vi "L298N stepper.vi"(2 "Baud Rate":u32=9600, 3 "Serial Port":refnum<visa-resource-name>) -> ()   [LabVIEW 2010]
uses:
  <vilib>/Instr/_visa.llb/VISA Set IO Buffer Mask.ctl
  <vilib>/Instr/_visa.llb/VISA Configure Serial Port (Instr).vi
panel:
  in  "stop":bool
  in  "Send":bool=TRUE
  out "Butes Written":u32
  out "X Step Position":i16
  out "String sent to Arduino":string
  in  "X Steps Setpoint":i16
  out "Status":errorcluster
  out "VISA resource\n name out":refnum<visa-resource-name>
  # "Serial Settings"
  # "Debug"
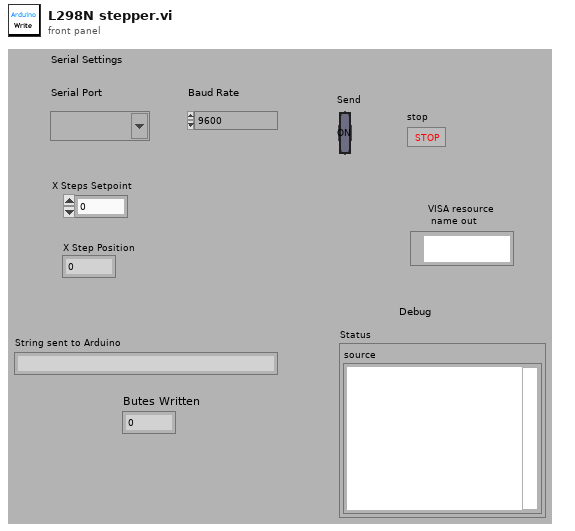
[diagram p1: front panel]
types:
  T1 = typedef "VISA Set IO Buffer Mask.ctl" = u16
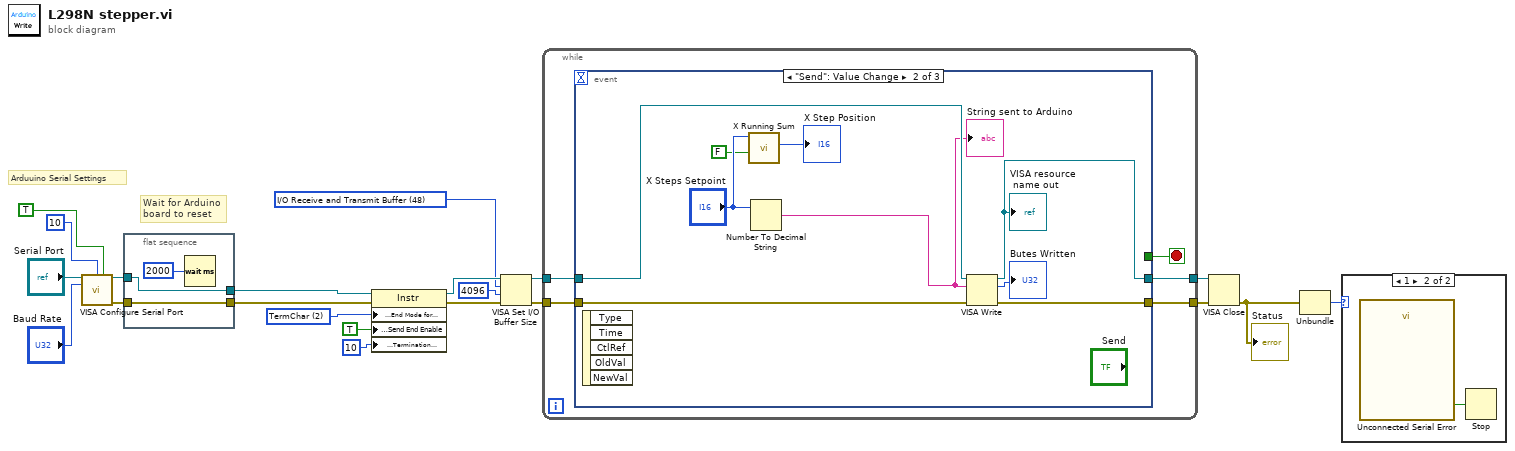
[diagram p0: block diagram]
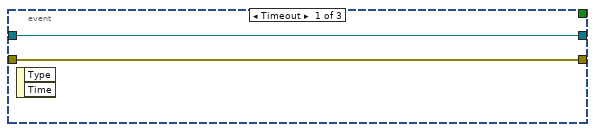
[diagram p2: hidden frame]
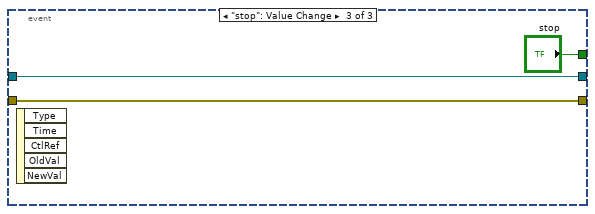
[diagram p3: hidden frame]
diagram:
  w7 = u16 2 items=["None", "Last Bit", "TermChar", "Break"] ("Serial Settings:End Mode for Writes")
  w5 = T1 48 items=["I/O Receive Buffer"=16, "I/O Transmit Buffer"=32, "I/O Receive and Transmit Buffer"=48] ("Mask")
  # "Wait for Arduino \nboard to reset"
  # "Arduuino Serial Settings"
  n1 = call-poly "VISA Configure Serial Port"("VISA resource name"="Serial Port", "termination char\n(0xA = '\\n' = LF)"=u8 10 ("termination char\n(0xA = '\\n' = LF)"), "Enable Termination\nChar (T)"=TRUE ("Enable Termination\nChar (T)"), "baud rate (9600)"="Baud Rate") -> ("VISA resource name out"=w15:refnum<visa-resource-name>, "error out"=w14:errorcluster)  [unwired: 10 in]
  n2 = flat-sequence {
    tunnel: [w24] -> w4
    tunnel: [w23] -> w3
    tunnel: w15 -> [w24]
    tunnel: w14 -> [w23]
    frame #0 {
      n3 = Wait (ms)(milliseconds to wait=u32 2000) -> ()  [unwired: 1 out]
    }
  }
  n4 = property class="Instr"(reference=w4, error in=w3, "Serial Settings:End Mode for Writes"=w7, "Message Based Settings:Send End Enable"=TRUE, "Message Based Settings:Termination Character"=u8 10) -> (reference out=w10:refnum<visa-resource-name>, error out=w11:errorcluster)
  n5 = VISA Set I/O Buffer Size(VISA resource name=w10, mask (16)=w5, size (4096)=u32 4096, error in (no error)=w11) -> (VISA resource name out=w2:refnum<visa-resource-name>, error out=w1:errorcluster)
  n6 = while {
    tunnel: [w29] -> w13
    tunnel: [w28] -> w12
    tunnel: w2 -> [w26]
    tunnel: w1 -> [w25]
    stop <- w27 stop-if-true
    n7 = event shown="[1] \"Send\": Value Change" {
      selector: _ -> [_ _ _]
      dyn-events: _ -> [_ _ _]
      timeout: _ -> [_ _ _]
      tunnel: w25 -> [w31 w40 w43]
      tunnel: [w31 w39 w43] -> w29
      tunnel: w26 -> [w30 w38 w42]
      tunnel: [w30 w36 w42] -> w28
      tunnel: [_ _ "stop"] -> w27
      event Timeout {
        n8 = event-data() -> ()  [unwired: 1 in, 2 out]
      }
      event "Send": Value Change {
        n9 = event-data() -> ()  [unwired: 1 in, 5 out]
        n10 = call "X Running Sum.vi"("Reset"=FALSE ("Send"), "X Input"="X Steps Setpoint") -> ("X Running Sum"=→"X Step Position":i16)  [unwired: 9 in]
        n11 = Number To Decimal String(number="X Steps Setpoint") -> (decimal integer string=w32:string)  [unwired: 1 in]
        "String sent to Arduino" <- w32
        n12 = VISA Write(VISA resource name=w38, write buffer=w32, error in (no error)=w40) -> (VISA resource name out=w36:refnum<visa-resource-name>, return count=→"Butes Written":u32, error out=w39:errorcluster)
        "VISA resource\n name out" <- w36
      }
      event "stop": Value Change {
        n13 = event-data() -> ()  [unwired: 1 in, 5 out]
      }
    }
  }
  n14 = VISA Close(VISA resource name=w12, error in (no error)=w13) -> (error out=w16:errorcluster)
  "Status" <- w16
  n15 = Unbundle(w16) -> ("code"=w17:i32)  [unwired: 2 out]
  n16 = case shown="1" w17 {
    frame 0, Default {
    }
    frame 1 {
      n17 = call "Unconnected Serial Error"() -> ("OK"=w44:bool)  [unwired: 10 in, 1 out]
      n18 = Stop(stop? (T)=w44) -> ()
    }
  }
